vi "Begin.vi"() -> (0 "error out":errorcluster)   [LabVIEW 2013]
doc: "Called before other user functions, this VI is expected to open initial I/O refnums, load in file data, and do all program initialization. Notice that the <B>error out</B> terminal is simply used for data flow. Wiring it to other structures or subVIs ensures that this VI runs first."
uses:
  <vilib>/Rock Robotics/WPI/Camera/WPI_CameraImageSize.ctl
  <vilib>/Rock Robotics/SystemInterfaces/DIO/FPGA_DIOPWMChannel.ctl
  <vilib>/Rock Robotics/WPI/SafetyOutput/WPI_SafetyOutputConfigMenu.ctl
  <vilib>/Rock Robotics/WPI/Joystick/WPI_JoystickDeviceEnum.ctl
  <vilib>/Rock Robotics/SystemInterfaces/DIO/FPGA_DIOChannel.ctl
  <vilib>/Rock Robotics/SystemInterfaces/Typedef/FPGA_TypedefAnalogModule.ctl
  <vilib>/Rock Robotics/SystemInterfaces/AI/FPGA_AIChannel.ctl
  <vilib>/Rock Robotics/SystemInterfaces/Typedef/FPGA_TypedefSolenoidModule.ctl
  <vilib>/Rock Robotics/WPI/Solenoid/WPI_SolenoidChannel.ctl
  <vilib>/Rock Robotics/WPI/Solenoid/WPI_SolenoidValue.ctl
  <vilib>/Rock Robotics/SystemInterfaces/Typedef/FPGA_TypedefDigitalModule.ctl
  <vilib>/Rock Robotics/SystemInterfaces/DIO/FPGA_DIORelayChannel.ctl
  <vilib>/Rock Robotics/WPI/Relay/WPI_RelayValue.ctl
  <vilib>/Rock Robotics/WPI/Relay/WPI_RelayDirection.ctl
  <vilib>/Rock Robotics/SystemInterfaces/Typedef/FPGA_TypedefAnalogModuleForGyro.ctl
  <vilib>/Rock Robotics/SystemInterfaces/AI/FPGA_AIGyroChannel.ctl
  <vilib>/Rock Robotics/WPI/DriverStation/WPI_DriverStationRobotMode2.ctl
  <vilib>/Rock Robotics/WPI/RobotDrive/WPI_RobotDriveOpen2MotorWithTalon.vi
  <vilib>/Rock Robotics/WPI/Counter/WPI_CounterDigitalInputToDigitalSource.vi
  <vilib>/Rock Robotics/WPI/Solenoid/WPI_SolenoidOpenDouble.vi
  <vilib>/Rock Robotics/WPI/Solenoid/WPI_SolenoidSetEnum.vi
  <vilib>/Rock Robotics/WPI/MotorControl/WPI_MotorControlOpen Victor.vi
  <vilib>/Rock Robotics/WPI/MotorControl/WPI_MotorControlOpen Talon.vi
  <vilib>/Rock Robotics/WPI/Counter/WPI_CounterOpen Gear Tooth Sensor Mode.vi
  Robot Global Data.vi
  <vilib>/Rock Robotics/WPI/Camera/WPI_CameraWhite Balance Values.ctl
  <vilib>/Rock Robotics/WPI/Camera/WPI_CameraExposure Values.ctl
  <vilib>/Rock Robotics/WPI/Camera/WPI_CameraFrameRate.ctl
  <vilib>/Rock Robotics/WPI/Counter/WPI_CounterOpen UpDown Mode.vi
  <vilib>/Rock Robotics/WPI/Solenoid/WPI_SolenoidOpenSingle.vi
panel:
  out "created new? axes":bool
  out "created new?":bool
  in  "Image Size":T1=enum."160x120"
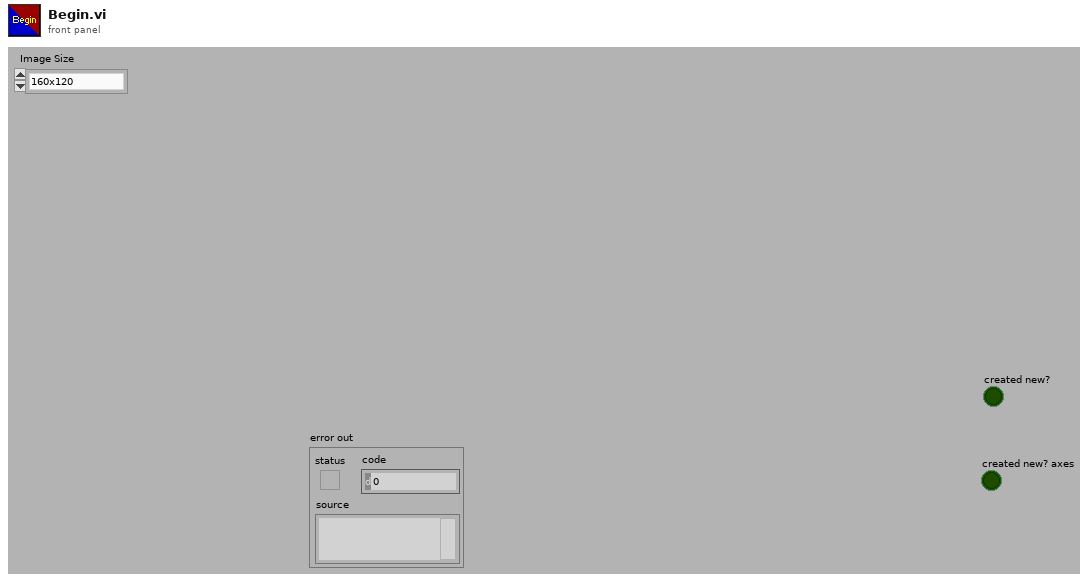
[diagram p1: front panel]
types:
  T1 = typedef "WPI_CameraImageSize.ctl" = enum16{"640x480", "320x240", "160x120"}
  T2 = typedef "WPI_DriverStationRobotMode2.ctl" = enum16{"Autonomous Disabled", "Autonomous Enabled", "Teleop Disabled", "Teleop Enabled", "Timeout", "Finish", "Test Disabled", "Test Enabled"}
  T3 = typedef "FPGA_AIChannel.ctl" = enum8{"AI 1", "AI 2", "AI 3", "AI 4", "AI 5", "AI 6", "AI 7", "AI 8", "Invalid"}
  T4 = typedef "FPGA_TypedefAnalogModule.ctl" = enum16{"Analog Module 1", "Analog Module 2"}
  T5 = typedef "FPGA_DIOPWMChannel.ctl" = enum8{"PWM 1", "PWM 2", "PWM 3", "PWM 4", "PWM 5", "PWM 6", "PWM 7", "PWM 8", "PWM 9", "PWM 10", "Invalid"}
  T6 = typedef "FPGA_TypedefDigitalModule.ctl" = enum16{"Digital Module 1", "Digital Module 2"}
  T7 = typedef "WPI_SolenoidValue.ctl" = enum16{"Off", "On", "Forward", "Reverse"}
  T8 = typedef "WPI_SolenoidChannel.ctl" = enum8{"Solenoid 1", "Solenoid 2", "Solenoid 3", "Solenoid 4", "Solenoid 5", "Solenoid 6", "Solenoid 7", "Solenoid 8", "Invalid"}
  T9 = typedef "FPGA_TypedefSolenoidModule.ctl" = enum16{"Solenoid Module 1", "Solenoid Module 2"}
  T10 = typedef "FPGA_DIOChannel.ctl" = enum8{"DIO 1", "DIO 2", "DIO 3", "DIO 4", "DIO 5", "DIO 6", "DIO 7", "DIO 8", "DIO 9", "DIO 10", "DIO 11", "DIO 12", "DIO 13", "DIO 14", "Invalid"}
  T11 = enum16{"open", "open or create", "create or replace", "create", "open (read-only)"}
  T12 = typedef "WPI_RelayDirection.ctl" = enum16{"Both directions", "Forward only", "Reverse only"}
  T13 = typedef "FPGA_DIORelayChannel.ctl" = enum8{"Relay 1", "Relay 2", "Relay 3", "Relay 4", "Relay 5", "Relay 6", "Relay 7", "Relay 8", "Invalid"}
  T14 = typedef "FPGA_AIGyroChannel.ctl" = enum8{"AI 1", "AI 2", "Invalid"}
  T15 = typedef "FPGA_TypedefAnalogModuleForGyro.ctl" = enum16{"Analog Module 1"}
  T16 = typedef "WPI_RelayValue.ctl" = enum16{"Off", "On", "Forward", "Reverse"}
  T17 = typedef "WPI_JoystickDeviceEnum.ctl" = enum16{"USB 1", "USB 2", "USB 3", "USB 4", "Kinect 1", "Kinect 2"}
  T18 = typedef "WPI_SafetyOutputConfigMenu.ctl" = enum16{"Enable", "Disable"}
  T19 = typedef "WPI_DigitalInputDevRef.ctl" = cluster{"DevStatus":errorcluster, "DIO Channel":T10, "Digital Module":T6}
  T20 = typedef "WPI_JoystickDevRef.ctl" = cluster{"Device":T17}
  T21 = typedef "WPI_RelayDevRef.ctl" = cluster{"DevStatus":errorcluster, "Relay Channel":T13, "Digital Module":T6, "Relay Direction":T12}
  T22 = enum16{"Rising Edge", "Falling Edge", "Raising & Falling Edge", "Disabled"}
  T23 = typedef "FPGA_CounterEncoderSourceConvertionLVSourceType.ctl" = cluster{"DevStatus":errorcluster, "AnalogTriggerMode?":bool, "DigitalMode":cluster{"Digital Module":T6, "DIO Channel":T24}, "AnalogTriggerMode":cluster{"AnalogTriggerIndex":T25, "OutputType":T26}}
  T24 = typedef "FPGA_DIODigitalSourceChannel.ctl" = enum8{"DIO 1", "DIO 2", "DIO 3", "DIO 4", "DIO 5", "DIO 6", "DIO 7", "DIO 8", "DIO 9", "DIO 10", "DIO 11", "DIO 12", "DIO 13", "DIO 14", "Disabled"}
  T25 = typedef "FPGA_AnalogTriggerIndex.ctl" = enum8{"Trig 0", "Trig 1", "Trig 2", "Trig 3", "Trig 4", "Trig 5", "Trig 6", "Trig 7", "Invalid"}
  T26 = typedef "FPGA_AnalogTriggerOutType.ctl" = enum16{"InWindow", "TriggerState", "Rising", "Falling"}
  T27 = typedef "WPI_CounterDevRef.ctl" = cluster{"DevStatus":errorcluster, "CntIndex":T28}
  T28 = typedef "FPGA_CounterCtrSystemIndex.ctl" = enum8{"Ctr 0", "Ctr 1", "Ctr 2", "Ctr 3", "Ctr 4", "Ctr 5", "Ctr 6", "Ctr 7", "Invalid"}
  T29 = typedef "WPI_ServoDeviceRef.ctl" = cluster{"DeviceStatus":errorcluster, "Digital Module":T6, "PWM Channel":T5, "DeadBand":T30}
  T30 = typedef "WPI_PWMDeadband.ctl" = cluster{"Name":string, "maxPositivePwm":i32, "minPositivePwm":i32, "centerPwm":i32, "maxNegativePwm":i32, "minNegativePwm":i32, "angularRange":u16}
  T31 = typedef "WPI_MotorControlDeviceRef.ctl" = cluster{"DeviceStatus":errorcluster, "Type":enum16{"PWM", "CAN"}, "PWM":cluster{"Digital Module":T6, "PWM Channel":T5, "DeadBand":T30}, "CAN":cluster{"Device Number":u8, "Control Mode":T32, "Semaphore":T33, "Max Vout":dbl}, "Invert":bool, "TransformRef":T34, "InvTransformRef":T34}
  T32 = typedef "WPI_CANJaguar_ControlMode.ctl" = enum8{"Percent VBus", "Current", "Speed", "Position", "Voltage"}
  T33 = typedef "Semaphore RefNum" = refnum<k1>
  T34 = typedef "WPI_PWMTransform_ConPane.ctl" = refnum<vi>
  T35 = typedef "WPI_SolenoidDevRef.ctl" = cluster{"DevStatus":errorcluster, "Solenoid Module":T9, "Forward Solenoid Channel":T8, "Reverse Solenoid Channel":T8}
  T36 = typedef "WPI_AnalogChannelDevRef.ctl" = cluster{"DevStatus":errorcluster, "Analog Module":T4, "Analog Channel":T3}
  T37 = typedef "WPI_RobotDriveDevRef.ctl" = cluster{"DevStatus":errorcluster, "Motors[]":T31[], "Square Inputs":bool, "Max Output":dbl, "Isochronous":bool}
  T38 = typedef "WPI_EncoderDevRef.ctl" = cluster{"DevStatus":errorcluster, "EncoderIndex":T39, "CounterIndex":T28, "DistancePerCount":dbl, "Decoding Type":T40}
  T39 = typedef "FPGA_EncoderIdx.ctl" = enum8{"Enc 0", "Enc 1", "Enc 2", "Enc 3", "Invalid"}
  T40 = typedef "WPI_EncoderType.ctl" = enum16{"1x", "2x", "4x"}
  T41 = typedef "WPI_GyroDevRef.ctl" = cluster{"DevStatus":errorcluster, "Analog Module":T4, "Analog Channel":T3, "Offset":dbl, "Gain (VoltsPerDegree/Second)":dbl}
  T42 = typedef "WPI_CameraFrameRate.ctl" = u32
  T43 = typedef "WPI_CameraExposure Values.ctl" = enum16{"Auto", "Flicker-free 50 Hz", "Flicker-free 60 Hz", "Hold current"}
  T44 = typedef "WPI_CameraWhite Balance Values.ctl" = enum16{"Auto", "Fixed indoor", "Fixed outdoor 1", "Fixed outdoor 2", "Fixed fluorescent 1", "Fixed fluorescent 2", "Hold current"}
  T45 = typedef "WPI_CameraDevRef.ctl" = cluster{"Camera Address":string, "CameraStatus":errorcluster, "Acquire Image Notifier":refnum<notifier>}
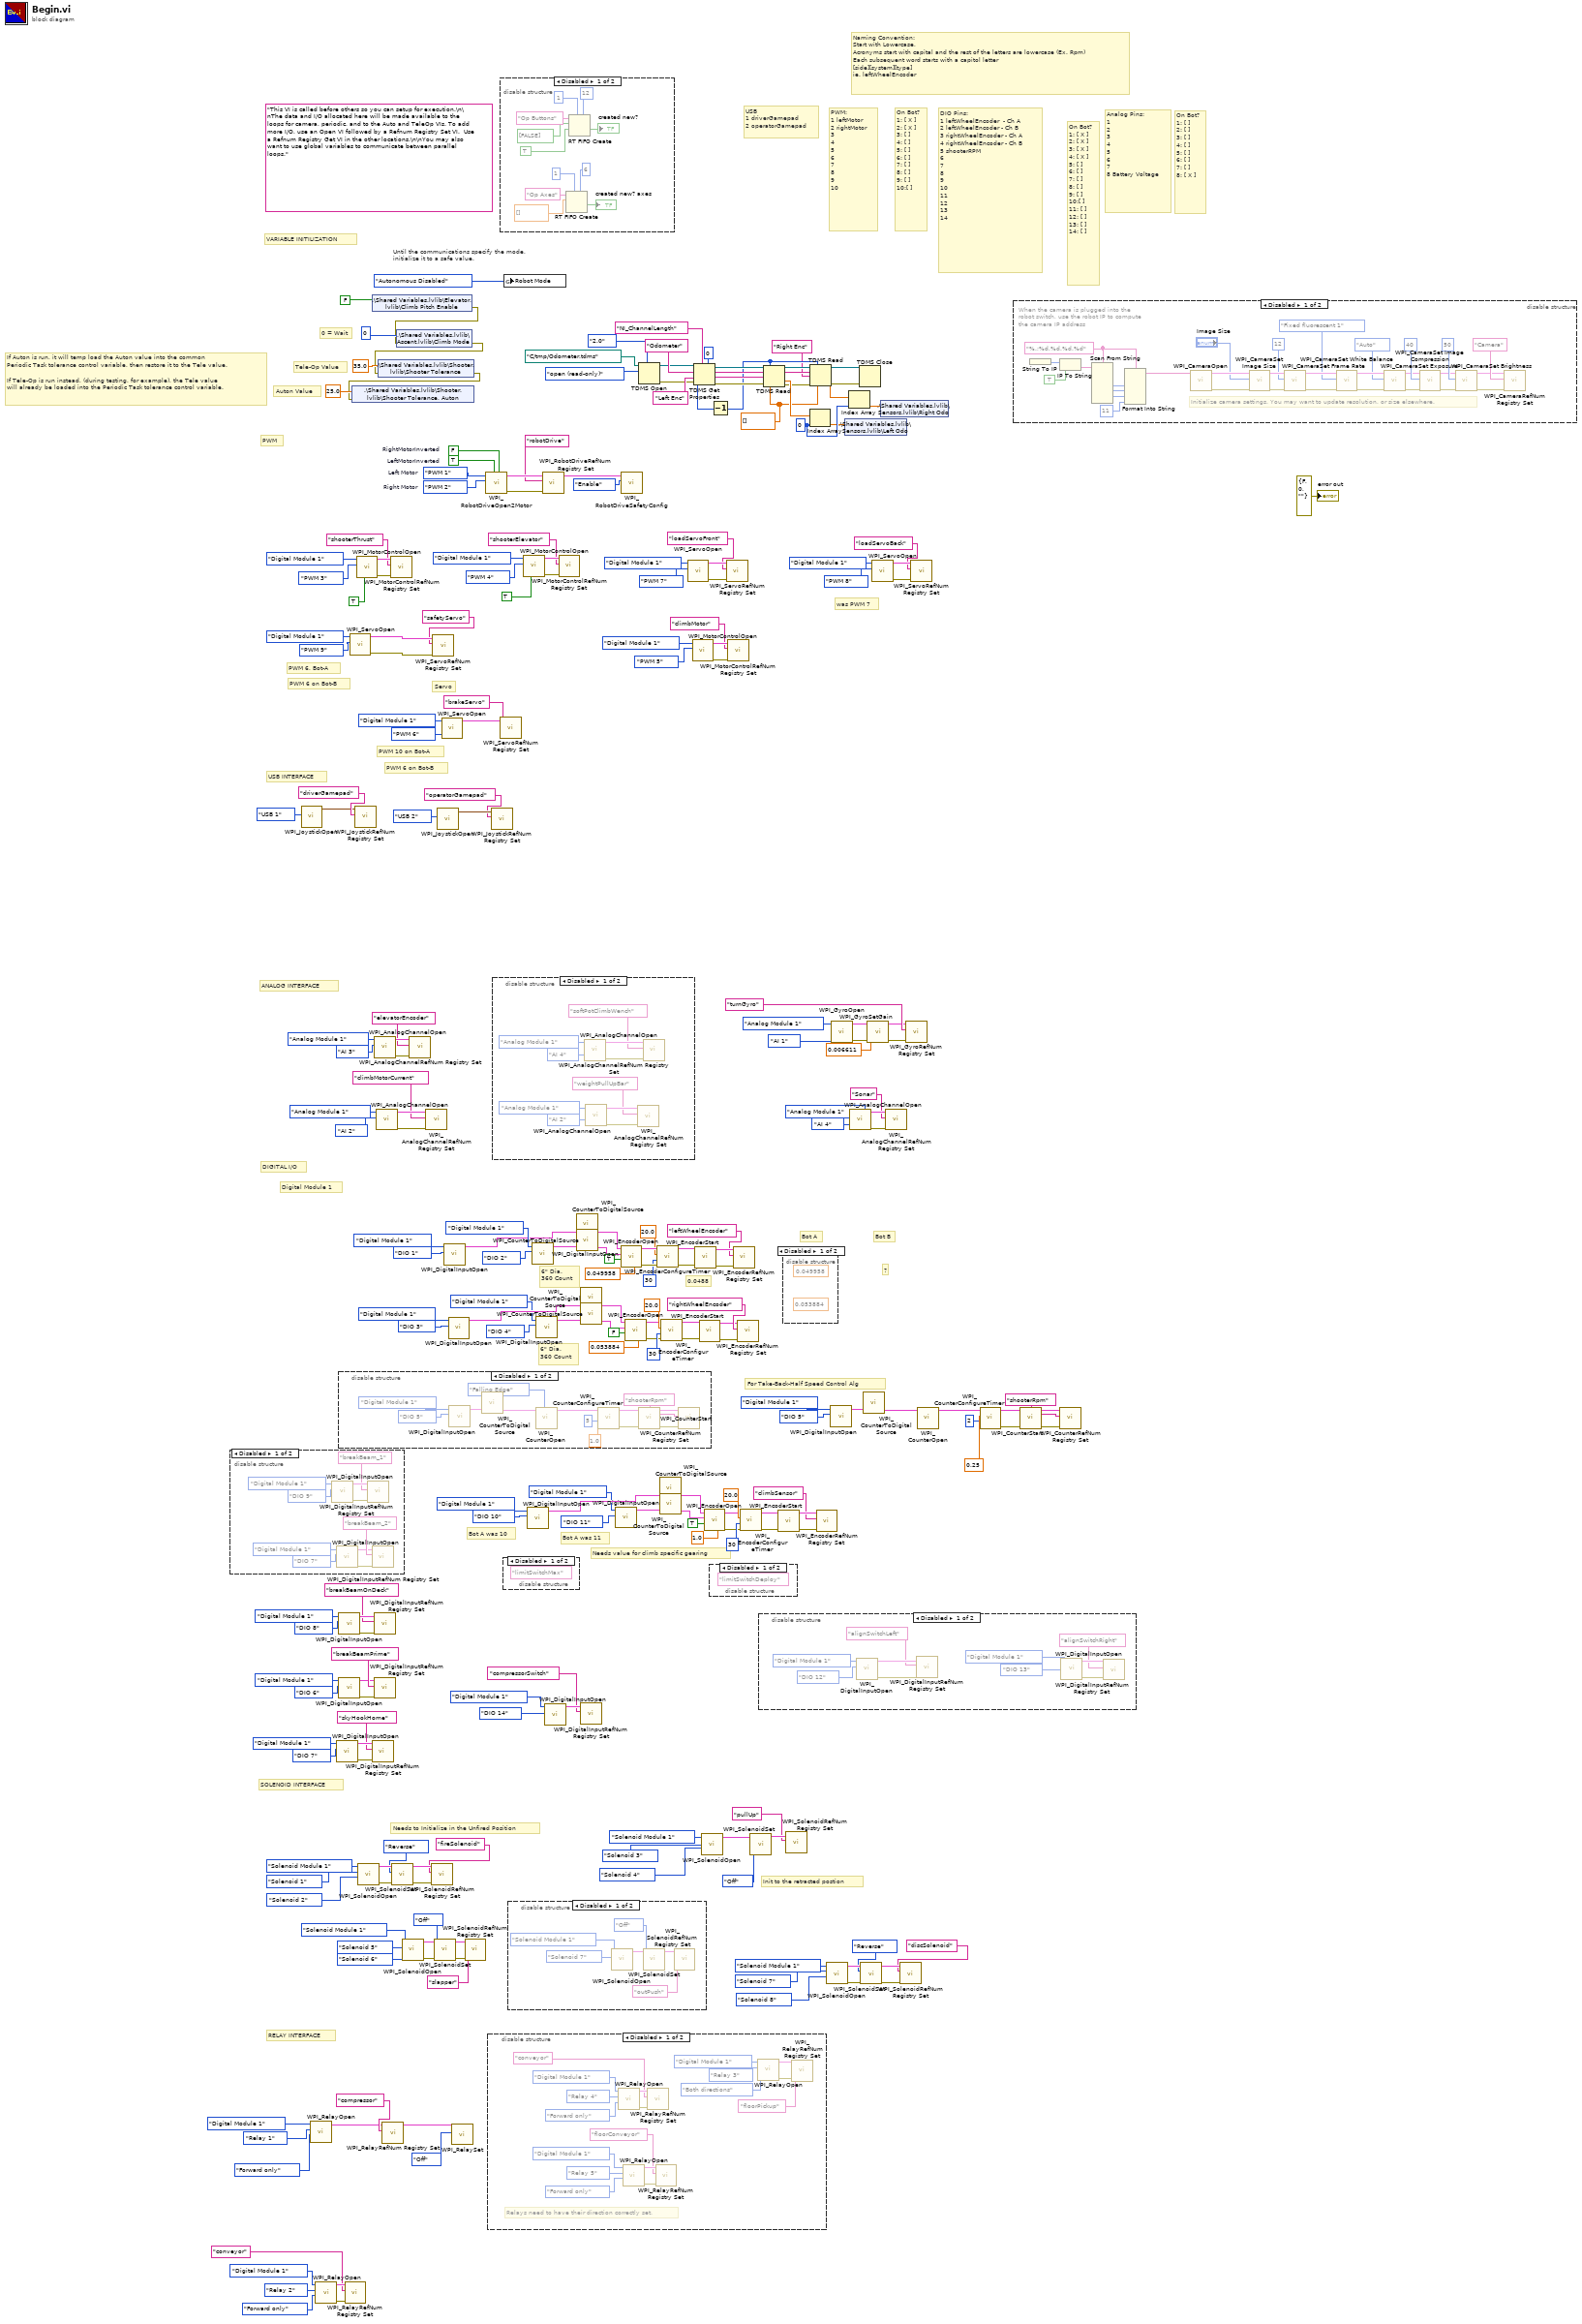
[diagram p0: block diagram]
diagram:
  w8 = 0 ("index")
  w12 = dbl[] []
  (unwired) "This VI is called before others so you can setup for execution.\n\nThe data and I/O allocated here will be made available to the loops for camera, periodic, and to the Auto and TeleOp VIs. To add more I/O, use an Open VI followed by a Refnum Registry Set VI.  Use a Refnum Registry Get VI in the other locations.\n\nYou may also want to use global variables to communicate between parallel loops."
  w239 = FPGA_DIOPWMChannel."PWM 2"  # Right Motor
  w240 = FPGA_DIOPWMChannel."PWM 1"  # Left Motor
  w244 = TRUE  # LeftMotorInverted
  w245 = FALSE  # RightMotorInverted
  # "If Auton is run, it will temp load the Auton value into the common\nPeriodic Task tolerance control variable, then restore it to the Tele value.\n\nIf Tele-Op is run instead, (during testing, for example), the Tele value\nwill already be loaded into the Periodic Task tolerance control variable."
  # "Auton Value"
  # "Tele-Op Value"
  # "Until the communications specify the mode,\ninitialize it to a safe value."
  # "0 = Wait"
  # "was PWM 7"
  # "PWM 10 on Bot-A"
  # "PWM 6 on Bot-B"
  # "PWM 6 on Bot-B"
  # "PWM 6, Bot-A"
  # "Servo"
  # "Bot A was 11"
  # "Bot A was 10"
  # "For Take-Back-Half Speed Control Alg"
  # "?"
  # "Bot B"
  # "Bot A"
  # "0.0488"
  # "Init to the retracted postion"
  # "Needs value for climb specific gearing"
  # "Needs to Initialize in the Unfired Position"
  # "Naming Convention:\nStart with Lowercase,\nAcronyms start with capital and the rest of the letters are lowercase (Ex. Rpm)\nEach subsequent word starts with a capitol letter\n[side][system][type]\nie. leftWheelEncoder"
  # "On Bot?\n1: [ ]\n2: [ ]\n3: [ ]\n4: [ ]\n5: [ ]\n6: [ ]\n7: [ ]\n8: [ X ]"
  # "On Bot?\n1: [ X ]\n2: [ X ]\n3: [ X ]\n4: [ X ]\n5: [ ]\n6: [ ]\n7: [ ]\n8: [ ]\n9: [ ]\n10:[ ]\n11: [ ]\n12: [ ]\n13: [ ]\n14: [ ]"
  # "On Bot?\n1: [ X ]\n2: [ X ]\n3: [ ]\n4: [ ]\n5: [ ]\n6: [ ]\n7: [ ]\n8: [ ]\n9: [ ]\n10:[ ]"
  # "6\" Dia. \n360 Count"
  # "6\" Dia. \n360 Count"
  # "PWM:\n1 leftMotor \n2 rightMotor\n3 \n4 \n5 \n6 \n7 \n8 \n9 \n10"
  # "USB\n1 driverGamepad\n2 operatorGamepad"
  # "Analog Pins:\n1 \n2 \n3 \n4 \n5 \n6 \n7 \n8 Battery Voltage"
  # "DIO Pins:\n1 leftWheelEncoder  - Ch A \n2 leftWheelEncoder - Ch B\n3 rightWheelEncoder - Ch A\n4 rightWheelEncoder - Ch B\n5 shooterRPM\n6  \n7 \n8 \n9 \n10 \n11 \n12 \n13 \n14"
  # "SOLENOID INTERFACE"
  # "Digital Module 1"
  # "DIGITAL I/O"
  # "ANALOG INTERFACE"
  # "RELAY INTERFACE"
  # "USB INTERFACE"
  # "VARIABLE INITILIZATION"
  # "PWM"
  n1 = disable-structure shown="Disabled" {
    frame Disabled {
      n2 = call <vilib>:"WPI_DigitalInputOpen.vi"("DIO Channel"=FPGA_DIOChannel."DIO 9", "Digital Module (Module 1)"=FPGA_TypedefDigitalModule."Digital Module 1") -> ("error out"=w255:errorcluster, "DigitalInputDevRef"=w254:T19)  [unwired: 8 in]
      n3 = call <vilib>:"WPI_DigitalInputOpen.vi"("DIO Channel"=FPGA_DIOChannel."DIO 7", "Digital Module (Module 1)"=FPGA_TypedefDigitalModule."Digital Module 1") -> ("error out"=w246:errorcluster, "DigitalInputDevRef"=w247:T19)  [unwired: 8 in]
      n4 = call <vilib>:"WPI_DigitalInputRefNum Registry Set.vi"("error in (no error)"=w255, "refnum name"="breakBeam_1", "DigitalInputDevRef"=w254) -> ()  [unwired: 7 in, 2 out]
      n5 = call <vilib>:"WPI_DigitalInputRefNum Registry Set.vi"("error in (no error)"=w246, "refnum name"="breakBeam_2", "DigitalInputDevRef"=w247) -> ()  [unwired: 7 in, 2 out]
    }
    frame Enabled {
    }
  }
  n6 = call <vilib>:"WPI_JoystickOpen.vi"("JoystickDevice"=WPI_JoystickDeviceEnum."USB 1") -> ("JoystickDevRef"=w235:T20)  [unwired: 10 in]
  n7 = call <vilib>:"WPI_RelayOpen.vi"("Relay Direction"=WPI_RelayDirection."Forward only", "Relay Channel"=FPGA_DIORelayChannel."Relay 1", "Digital Module (Module 1)"=FPGA_TypedefDigitalModule."Digital Module 1" ("Relay Digital Module (Module 1)")) -> ("RelayDevRef"=w100:T21)  [unwired: 7 in, 1 out]
  n8 = call <vilib>:"WPI_RelayOpen.vi"("Relay Direction"=WPI_RelayDirection."Forward only", "Relay Channel"=FPGA_DIORelayChannel."Relay 2", "Digital Module (Module 1)"=FPGA_TypedefDigitalModule."Digital Module 1") -> ("error out"=w86:errorcluster, "RelayDevRef"=w85:T21)  [unwired: 7 in]
  n9 = call <vilib>:"WPI_DigitalInputOpen.vi"("DIO Channel"=FPGA_DIOChannel."DIO 7", "Digital Module (Module 1)"=FPGA_TypedefDigitalModule."Digital Module 1") -> ("error out"=w55:errorcluster, "DigitalInputDevRef"=w54:T19)  [unwired: 8 in]
  n10 = disable-structure shown="Disabled" {
    frame Disabled {
      n11 = call <vilib>:"WPI_DigitalInputOpen.vi"("DIO Channel"=FPGA_DIOChannel."DIO 5", "Digital Module (Module 1)"=FPGA_TypedefDigitalModule."Digital Module 1") -> ("DigitalInputDevRef"=w268:T19)  [unwired: 8 in, 1 out]
      n12 = call-poly <vilib>:"WPI_CounterToDigitalSource.vi"("DigitalInputDevRef"=w268) -> ("Digital Source"=w267:T23)  [unwired: 6 in]
      n13 = call-poly <vilib>:"WPI_CounterOpen.vi"("UpEdge"=T22."Falling Edge", "Up Source"=w267) -> ("CounterDevRef"=w263:T27)  [unwired: 8 in, 1 out]
      n14 = call <vilib>:"WPI_CounterConfigureTimer.vi"("Number Samples to Average"=u8 5, "MaxPeriod (sec)"=1.0, "CounterDevRef in"=w263) -> ("error out"=w260:errorcluster, "CounterDevRef out"=w259:T27)  [unwired: 7 in]
      n15 = call <vilib>:"WPI_CounterStart.vi"("error in (no error)"=w260, "CounterDevRef in"=w259) -> ("error out"=w258:errorcluster, "CounterDevRef out"=w257:T27)  [unwired: 8 in]
      n16 = call <vilib>:"WPI_CounterRefNum Registry Set.vi"("error in (no error)"=w258, "refnum name"="shooterRpm", "CounterDevRef"=w257) -> ()  [unwired: 7 in, 2 out]
    }
    frame Enabled {
    }
  }
  n17 = call <vilib>:"WPI_DigitalInputOpen.vi"("DIO Channel"=FPGA_DIOChannel."DIO 8", "Digital Module (Module 1)"=FPGA_TypedefDigitalModule."Digital Module 1") -> ("error out"=w186:errorcluster, "DigitalInputDevRef"=w185:T19)  [unwired: 8 in]
  n18 = call <vilib>:"WPI_DigitalInputOpen.vi"("DIO Channel"=FPGA_DIOChannel."DIO 6", "Digital Module (Module 1)"=FPGA_TypedefDigitalModule."Digital Module 1") -> ("error out"=w177:errorcluster, "DigitalInputDevRef"=w178:T19)  [unwired: 8 in]
  n19 = call <vilib>:"WPI_RelayRefNum Registry Set.vi"("error in (no error)"=w86, "refnum name"="conveyor", "RelayDevRef"=w85) -> ()  [unwired: 7 in, 2 out]
  n20 = call <vilib>:"WPI_ServoOpen.vi"("PWM Channel"=FPGA_DIOPWMChannel."PWM 9", "Digital Module (Module 1)"=FPGA_TypedefDigitalModule."Digital Module 1") -> ("error out"=w161:errorcluster, "ServoDeviceRef"=w162:T29)  [unwired: 8 in]
  n21 = call <vilib>:"WPI_JoystickRefNum Registry Set.vi"("refnum name"="driverGamepad", "JoystickDevRef"=w235) -> ()  [unwired: 8 in, 2 out]
  n22 = call-poly <vilib>:"WPI_MotorControlOpen.vi"("Invert"=TRUE, "PWM Channel"=FPGA_DIOPWMChannel."PWM 3", "Digital Module (Module 1)"=FPGA_TypedefDigitalModule."Digital Module 1") -> ("error out"=w156:errorcluster, "MotorControlDeviceRef"=w157:T31)  [unwired: 7 in]
  n23 = call-poly <vilib>:"WPI_SolenoidOpen.vi"("Reverse Solenoid Channel"=WPI_SolenoidChannel."Solenoid 2", "Forward Solenoid Channel"=WPI_SolenoidChannel."Solenoid 1", "Solenoid Module (Module 1)"=FPGA_TypedefSolenoidModule."Solenoid Module 1") -> ("error out"=w173:errorcluster, "SolenoidDevRef"=w172:T35)  [unwired: 7 in]
  n24 = call <vilib>:"WPI_DigitalInputRefNum Registry Set.vi"("error in (no error)"=w55, "refnum name"="skyHookHome", "DigitalInputDevRef"=w54) -> ()  [unwired: 7 in, 2 out]
  n25 = shared-variable ".\\Shared Variables.lvlib\\Elevator.lvlib\\Climb Pitch Enable"(FALSE ("Climb Pitch Enable")) -> (error out=w5:errorcluster)  [unwired: 1 in]
  n26 = call <vilib>:"WPI_AnalogChannelOpen.vi"("Analog Channel"=FPGA_AIChannel."AI 3", "Analog Module (Module 1)"=FPGA_TypedefAnalogModule."Analog Module 1") -> ("error out"=w189:errorcluster, "AIDeviceRef"=w188:T36)  [unwired: 8 in]
  n27 = call <vilib>:"WPI_DigitalInputRefNum Registry Set.vi"("error in (no error)"=w186, "refnum name"="breakBeamOnDeck", "DigitalInputDevRef"=w185) -> ()  [unwired: 7 in, 2 out]
  n28 = call <vilib>:"WPI_DigitalInputRefNum Registry Set.vi"("error in (no error)"=w177, "refnum name"="breakBeamPrime", "DigitalInputDevRef"=w178) -> ()  [unwired: 7 in, 2 out]
  n29 = call <vilib>:"WPI_AnalogChannelOpen.vi"("Analog Channel"=FPGA_AIChannel."AI 2", "Analog Module (Module 1)"=FPGA_TypedefAnalogModule."Analog Module 1") -> ("error out"=w146:errorcluster, "AIDeviceRef"=w147:T36)  [unwired: 8 in]
  n30 = call <vilib>:"WPI_RelayRefNum Registry Set.vi"("refnum name"="compressor", "RelayDevRef"=w100) -> ("RelayDevRef"=w99:T21)  [unwired: 8 in, 1 out]
  n31 = call <vilib>:"WPI_MotorControlRefNum Registry Set.vi"("error in (no error)"=w156, "refnum name"="shooterThrust", "MotorControlDevRef"=w157) -> ()  [unwired: 7 in, 2 out]
  n32 = call-poly <vilib>:"WPI_SolenoidSet.vi"("error in (no error)"=w173, "Value"=WPI_SolenoidValue."Reverse", "SolenoidDevRef"=w172) -> ("error out"=w170:errorcluster, "SolenoidDevRef"=w169:T35)  [unwired: 7 in]
  n33 = shared-variable ".\\Shared Variables.lvlib\\Ascent.lvlib\\Climb Mode"(u16 0 ("Climb Mode"), error in=w5) -> (error out=w2:errorcluster)
  n34 = shared-variable ".\\Shared Variables.lvlib\\Shooter.lvlib\\Shooter Tolerance"(35.0 ("Shooter Tolerance"), error in=w2) -> (error out=w1:errorcluster)
  n35 = shared-variable ".\\Shared Variables.lvlib\\Shooter.lvlib\\Shooter Tolerance, Auton"(25.0 ("Shooter Tolerance, Auton"), error in=w1) -> ()  [unwired: 1 out]
  n36 = call-poly <vilib>:"WPI_SolenoidOpen.vi"("Reverse Solenoid Channel"=WPI_SolenoidChannel."Solenoid 6", "Forward Solenoid Channel"=WPI_SolenoidChannel."Solenoid 5", "Solenoid Module (Module 1)"=FPGA_TypedefSolenoidModule."Solenoid Module 1") -> ("error out"=w142:errorcluster, "SolenoidDevRef"=w141:T35)  [unwired: 7 in]
  n37 = call <vilib>:"WPI_AnalogChannelRefNum Registry Set.vi"("error in (no error)"=w189, "refnum name"="elevatorEncoder", "AIDeviceRef"=w188) -> ()  [unwired: 7 in, 2 out]
  n38 = call <vilib>:"WPI_AnalogChannelRefNum Registry Set.vi"("error in (no error)"=w146, "refnum name"="climbMotorCurrent", "AIDeviceRef"=w147) -> ()  [unwired: 7 in, 2 out]
  n39 = call <vilib>:"WPI_SolenoidRefNum Registry Set.vi"("error in (no error)"=w170, "refnum name"="fireSolenoid", "SolenoidDevRef"=w169) -> ()  [unwired: 7 in, 2 out]
  n40 = call <vilib>:"WPI_ServoRefNum Registry Set.vi"("error in (no error)"=w161, "refnum name"="safetyServo", "ServoDeviceRef"=w162) -> ()  [unwired: 7 in, 2 out]
  n41 = call-poly <vilib>:"WPI_SolenoidSet.vi"("error in (no error)"=w142, "Value"=WPI_SolenoidValue."Off", "SolenoidDevRef"=w141) -> ("error out"=w140:errorcluster, "SolenoidDevRef"=w139:T35)  [unwired: 7 in]
  n42 = call <vilib>:"WPI_JoystickOpen.vi"("JoystickDevice"=WPI_JoystickDeviceEnum."USB 2") -> ("JoystickDevRef"=w194:T20)  [unwired: 10 in]
  n43 = call <vilib>:"WPI_ServoOpen.vi"("PWM Channel"=FPGA_DIOPWMChannel."PWM 6", "Digital Module (Module 1)"=FPGA_TypedefDigitalModule."Digital Module 1") -> ("ServoDeviceRef"=w27:T29)  [unwired: 8 in, 1 out]
  n44 = call <vilib>:"WPI_DigitalInputOpen.vi"("DIO Channel"=FPGA_DIOChannel."DIO 1", "Digital Module (Module 1)"=FPGA_TypedefDigitalModule."Digital Module 1") -> ("DigitalInputDevRef"=w228:T19)  [unwired: 8 in, 1 out]
  n45 = call <vilib>:"WPI_DigitalInputOpen.vi"("DIO Channel"=FPGA_DIOChannel."DIO 3", "Digital Module (Module 1)"=FPGA_TypedefDigitalModule."Digital Module 1") -> ("DigitalInputDevRef"=w201:T19)  [unwired: 8 in, 1 out]
  n46 = call <vilib>:"WPI_RelaySet.vi"("RelayValue"=WPI_RelayValue."Off", "RelayDevRef"=w99) -> ()  [unwired: 8 in, 2 out]
  n47 = call <vilib>:"WPI_SolenoidRefNum Registry Set.vi"("error in (no error)"=w140, "refnum name"="slapper", "SolenoidDevRef"=w139) -> ()  [unwired: 7 in, 2 out]
  n48 = call-poly <vilib>:"WPI_RobotDriveOpen2Motor.vi"("Right Motor Inverted"=w245, "Left Motor Inverted"=w244, "Right Motor"=w239, "Left Motor"=w240) -> ("error out"=w241:errorcluster, "RobotDriveDevRef"=w243:T37)  [unwired: 6 in]
  n49 = disable-structure shown="Disabled" {
    frame Disabled {
      # "Relays need to have their direction correctly set."
      n50 = call <vilib>:"WPI_RelayOpen.vi"("Relay Direction"=WPI_RelayDirection."Forward only", "Relay Channel"=FPGA_DIORelayChannel."Relay 4", "Digital Module (Module 1)"=FPGA_TypedefDigitalModule."Digital Module 1") -> ("error out"=w286:errorcluster, "RelayDevRef"=w285:T21)  [unwired: 7 in]
      n51 = call <vilib>:"WPI_RelayOpen.vi"("Relay Direction"=WPI_RelayDirection."Forward only", "Relay Channel"=FPGA_DIORelayChannel."Relay 5", "Digital Module (Module 1)"=FPGA_TypedefDigitalModule."Digital Module 1") -> ("error out"=w280:errorcluster, "RelayDevRef"=w279:T21)  [unwired: 7 in]
      n52 = call <vilib>:"WPI_RelayRefNum Registry Set.vi"("error in (no error)"=w286, "refnum name"="conveyor", "RelayDevRef"=w285) -> ()  [unwired: 7 in, 2 out]
      n53 = call <vilib>:"WPI_RelayRefNum Registry Set.vi"("error in (no error)"=w280, "refnum name"="floorConveyor", "RelayDevRef"=w279) -> ()  [unwired: 7 in, 2 out]
      n54 = call <vilib>:"WPI_RelayOpen.vi"("Relay Direction"=WPI_RelayDirection."Both directions", "Relay Channel"=FPGA_DIORelayChannel."Relay 3", "Digital Module (Module 1)"=FPGA_TypedefDigitalModule."Digital Module 1") -> ("error out"=w273:errorcluster, "RelayDevRef"=w274:T21)  [unwired: 7 in]
      n55 = call <vilib>:"WPI_RelayRefNum Registry Set.vi"("error in (no error)"=w273, "refnum name"="floorPickup", "RelayDevRef"=w274) -> ()  [unwired: 7 in, 2 out]
    }
    frame Enabled {
    }
  }
  n56 = call <vilib>:"WPI_JoystickRefNum Registry Set.vi"("refnum name"="operatorGamepad", "JoystickDevRef"=w194) -> ()  [unwired: 8 in, 2 out]
  n57 = disable-structure shown="Disabled" {
    frame Disabled {
      n58 = call <vilib>:"WPI_AnalogChannelOpen.vi"("Analog Channel"=FPGA_AIChannel."AI 4", "Analog Module (Module 1)"=FPGA_TypedefAnalogModule."Analog Module 1") -> ("error out"=w295:errorcluster, "AIDeviceRef"=w296:T36)  [unwired: 8 in]
      n59 = call <vilib>:"WPI_AnalogChannelOpen.vi"("Analog Channel"=FPGA_AIChannel."AI 2", "Analog Module (Module 1)"=FPGA_TypedefAnalogModule."Analog Module 1") -> ("error out"=w293:errorcluster, "AIDeviceRef"=w294:T36)  [unwired: 8 in]
      n60 = call <vilib>:"WPI_AnalogChannelRefNum Registry Set.vi"("error in (no error)"=w293, "refnum name"="weightPullUpBar", "AIDeviceRef"=w294) -> ()  [unwired: 7 in, 2 out]
      n61 = call <vilib>:"WPI_AnalogChannelRefNum Registry Set.vi"("error in (no error)"=w295, "refnum name"="softPotClimbWench", "AIDeviceRef"=w296) -> ()  [unwired: 7 in, 2 out]
    }
    frame Enabled {
    }
  }
  n62 = disable-structure shown="Disabled" {
    frame Disabled {
      n63 = RT FIFO Create(0:"Op Axes" ("name (unnamed)"), 1:dbl[] [], 4:u32 1 ("size (10)"), 6:u32 6 ("elements in array (1)")) -> (10:→"created new? axes":bool)  [unwired: 4 in, 2 out]
      n64 = RT FIFO Create(0:"Op Buttons" ("name (unnamed)"), 1:bool[] [FALSE], 2:TRUE ("create if not found? (T)"), 4:u32 1 ("size (10)"), 6:u32 12 ("elements in array (1)")) -> (10:→"created new?":bool)  [unwired: 3 in, 2 out]
    }
    frame Enabled {
    }
  }
  n65 = call <vilib>:"WPI_ServoRefNum Registry Set.vi"("refnum name"="brakeServo", "ServoDeviceRef"=w27) -> ()  [unwired: 8 in, 2 out]
  n66 = disable-structure shown="Disabled" {
    frame Disabled {
      (unwired) "limitSwitchMax" ("refnum name")
    }
    frame Enabled {
    }
  }
  n67 = global write "Robot Global Data.vi" "Robot Mode"(WPI_DriverStationRobotMode2."Autonomous Disabled" ("Robot Mode")) -> ()
  n68 = disable-structure shown="Disabled" {
    frame Disabled {
      n69 = call-poly <vilib>:"WPI_SolenoidOpen.vi"("Solenoid Channel"=WPI_SolenoidChannel."Solenoid 7" ("Forward Solenoid Channel"), "Solenoid Module (Module 1)"=FPGA_TypedefSolenoidModule."Solenoid Module 1") -> ("SolenoidDevRef"=w313:T35)  [unwired: 8 in, 1 out]
      n70 = call-poly <vilib>:"WPI_SolenoidSet.vi"("Value"=WPI_SolenoidValue."Off", "SolenoidDevRef"=w313) -> ("SolenoidDevRef"=w312:T35)  [unwired: 8 in, 1 out]
      n71 = call <vilib>:"WPI_SolenoidRefNum Registry Set.vi"("refnum name"="outPush", "SolenoidDevRef"=w312) -> ()  [unwired: 8 in, 2 out]
    }
    frame Enabled {
    }
  }
  n72 = call-poly <vilib>:"WPI_MotorControlOpen.vi"("Invert"=TRUE, "PWM Channel"=FPGA_DIOPWMChannel."PWM 4", "Digital Module (Module 1)"=FPGA_TypedefDigitalModule."Digital Module 1") -> ("error out"=w154:errorcluster, "MotorControlDeviceRef"=w155:T31)  [unwired: 7 in]
  n73 = call <vilib>:"WPI_DigitalInputOpen.vi"("DIO Channel"=FPGA_DIOChannel."DIO 10", "Digital Module (Module 1)"=FPGA_TypedefDigitalModule."Digital Module 1") -> ("DigitalInputDevRef"=w122:T19)  [unwired: 8 in, 1 out]
  n74 = call <vilib>:"WPI_DigitalInputOpen.vi"("DIO Channel"=FPGA_DIOChannel."DIO 2", "Digital Module (Module 1)"=FPGA_TypedefDigitalModule."Digital Module 1") -> ("DigitalInputDevRef"=w229:T19)  [unwired: 8 in, 1 out]
  n75 = call <vilib>:"WPI_DigitalInputOpen.vi"("DIO Channel"=FPGA_DIOChannel."DIO 4", "Digital Module (Module 1)"=FPGA_TypedefDigitalModule."Digital Module 1") -> ("DigitalInputDevRef"=w200:T19)  [unwired: 8 in, 1 out]
  n76 = call <vilib>:"WPI_RobotDriveRefNum Registry Set.vi"("error in (no error)"=w241, "refnum name"="robotDrive", "RobotDriveDevRef"=w243) -> ("RobotDriveDevRef"=w238:T37)  [unwired: 8 out]
  n77 = call <vilib>:"WPI_DigitalInputOpen.vi"("DIO Channel"=FPGA_DIOChannel."DIO 14" ("Pressure Switch DIO Channel"), "Digital Module (Module 1)"=FPGA_TypedefDigitalModule."Digital Module 1" ("Pressure Switch Digital Module (Module 1)")) -> ("DigitalInputDevRef"=w92:T19)  [unwired: 8 in, 1 out]
  n78 = call <vilib>:"WPI_MotorControlRefNum Registry Set.vi"("error in (no error)"=w154, "refnum name"="shooterElevator", "MotorControlDevRef"=w155) -> ()  [unwired: 7 in, 2 out]
  n79 = call-poly <vilib>:"WPI_CounterToDigitalSource.vi"("DigitalInputDevRef"=w228) -> ("Digital Source"=w227:T23)  [unwired: 6 in]
  n80 = call-poly <vilib>:"WPI_CounterToDigitalSource.vi"("DigitalInputDevRef"=w229) -> ("Digital Source"=w226:T23)  [unwired: 6 in]
  n81 = call-poly <vilib>:"WPI_CounterToDigitalSource.vi"("DigitalInputDevRef"=w201) -> ("Digital Source"=w202:T23)  [unwired: 6 in]
  n82 = call-poly <vilib>:"WPI_CounterToDigitalSource.vi"("DigitalInputDevRef"=w200) -> ("Digital Source"=w203:T23)  [unwired: 6 in]
  n83 = call <vilib>:"WPI_DigitalInputRefNum Registry Set.vi"("refnum name"="compressorSwitch", "DigitalInputDevRef"=w92) -> ()  [unwired: 8 in, 2 out]
  n84 = call <vilib>:"WPI_DigitalInputOpen.vi"("DIO Channel"=FPGA_DIOChannel."DIO 11", "Digital Module (Module 1)"=FPGA_TypedefDigitalModule."Digital Module 1") -> ("DigitalInputDevRef"=w121:T19)  [unwired: 8 in, 1 out]
  n85 = call <vilib>:"WPI_EncoderOpen.vi"("DistancePerCount"=0.049958, "Invert Direction (False)"=TRUE, "BSource"=w226, "ASource"=w227) -> ("error out"=w223:errorcluster, "EncoderDevRef"=w222:T38)  [unwired: 6 in]
  n86 = call <vilib>:"WPI_RobotDriveSafetyConfig.vi"("mode"=WPI_SafetyOutputConfigMenu."Enable", "RobotDriveDevRef"=w238) -> ()  [unwired: 8 in, 2 out]
  n87 = call <vilib>:"WPI_EncoderOpen.vi"("DistancePerCount"=0.053884, "Invert Direction (False)"=FALSE, "BSource"=w203, "ASource"=w202) -> ("error out"=w206:errorcluster, "EncoderDevRef"=w207:T38)  [unwired: 6 in]
  n88 = TDMS Open(7:enum16{"1.0", "2.0"}."2.0" ("file format version (2.0)"), 10:T11."open (read-only)" ("operation (0:open)"), 11:path "C:/tmp/Odometer.tdms" ("file path")) -> (0:w67:errorcluster, 3:w65:refnum<k34>)  [unwired: 4 in]
  n89 = call <vilib>:"WPI_EncoderConfigureTimer.vi"("error in (no error)"=w223, "Number Samples to Average"=u8 30, "Minimum Rate"=20.0, "EncoderDevRef"=w222) -> ("error out"=w219:errorcluster, "EncoderDevRef"=w218:T38)  [unwired: 6 in]
  n90 = call-poly <vilib>:"WPI_CounterToDigitalSource.vi"("DigitalInputDevRef"=w122) -> ("Digital Source"=w123:T23)  [unwired: 6 in]
  n91 = call-poly <vilib>:"WPI_CounterToDigitalSource.vi"("DigitalInputDevRef"=w121) -> ("Digital Source"=w124:T23)  [unwired: 6 in]
  n92 = call <vilib>:"WPI_EncoderConfigureTimer.vi"("error in (no error)"=w206, "Number Samples to Average"=u8 30, "Minimum Rate"=20.0, "EncoderDevRef"=w207) -> ("error out"=w210:errorcluster, "EncoderDevRef"=w211:T38)  [unwired: 6 in]
  n93 = call <vilib>:"WPI_ServoOpen.vi"("PWM Channel"=FPGA_DIOPWMChannel."PWM 7", "Digital Module (Module 1)"=FPGA_TypedefDigitalModule."Digital Module 1") -> ("error out"=w167:errorcluster, "ServoDeviceRef"=w166:T29)  [unwired: 8 in]
  n94 = call-poly <vilib>:"WPI_MotorControlOpen.vi"("PWM Channel"=FPGA_DIOPWMChannel."PWM 5", "Digital Module (Module 1)"=FPGA_TypedefDigitalModule."Digital Module 1") -> ("error out"=w114:errorcluster, "MotorControlDeviceRef"=w115:T31)  [unwired: 8 in]
  n95 = TDMS Get Properties(5:0, 7:"NI_ChannelLength" ("property name"), 8:w67, 9:"Left Enc" ("channel name"), 10:"Odometer" ("group name"), 11:w65) -> (0:w66:errorcluster, 1:w70:string, 2:w71:string, 3:w69:refnum<k34>, 4:w64:i32)  [unwired: 1 out]
  n96 = call <vilib>:"WPI_EncoderStart.vi"("error in (no error)"=w219, "EncoderDevRef"=w218) -> ("error out"=w217:errorcluster, "EncoderDevRef"=w216:T38)  [unwired: 8 in]
  n97 = call <vilib>:"WPI_EncoderStart.vi"("error in (no error)"=w210, "EncoderDevRef"=w211) -> ("error out"=w212:errorcluster, "EncoderDevRef"=w213:T38)  [unwired: 8 in]
  n98 = call-poly <vilib>:"WPI_SolenoidOpen.vi"("Reverse Solenoid Channel"=WPI_SolenoidChannel."Solenoid 4", "Forward Solenoid Channel"=WPI_SolenoidChannel."Solenoid 3", "Solenoid Module (Module 1)"=FPGA_TypedefSolenoidModule."Solenoid Module 1") -> ("SolenoidDevRef"=w108:T35)  [unwired: 7 in, 1 out]
  n99 = call <vilib>:"WPI_EncoderOpen.vi"("DistancePerCount"=1.0, "Invert Direction (False)"=TRUE, "BSource"=w124, "ASource"=w123) -> ("error out"=w127:errorcluster, "EncoderDevRef"=w128:T38)  [unwired: 6 in]
  n100 = disable-structure shown="Disabled" {
    frame Disabled {
      (unwired) "limitSwitchDeploy" ("refnum name")
    }
    frame Enabled {
    }
  }
  n101 = Decrement(x=w64) -> (x-1=w63:i32)
  n102 = call <vilib>:"WPI_ServoRefNum Registry Set.vi"("error in (no error)"=w167, "refnum name"="loadServoFront", "ServoDeviceRef"=w166) -> ()  [unwired: 7 in, 2 out]
  n103 = call <vilib>:"WPI_MotorControlRefNum Registry Set.vi"("error in (no error)"=w114, "refnum name"="climbMotor", "MotorControlDevRef"=w115) -> ()  [unwired: 7 in, 2 out]
  n104 = call <vilib>:"WPI_EncoderRefNum Registry Set.vi"("error in (no error)"=w217, "refnum name"="leftWheelEncoder", "EncoderDevRef"=w216) -> ()  [unwired: 7 in, 2 out]
  n105 = call <vilib>:"WPI_EncoderRefNum Registry Set.vi"("error in (no error)"=w212, "refnum name"="rightWheelEncoder", "EncoderDevRef"=w213) -> ()  [unwired: 7 in, 2 out]
  n106 = call <vilib>:"WPI_EncoderConfigureTimer.vi"("error in (no error)"=w127, "Number Samples to Average"=u8 30, "Minimum Rate"=20.0, "EncoderDevRef"=w128) -> ("error out"=w131:errorcluster, "EncoderDevRef"=w132:T38)  [unwired: 6 in]
  n107 = call-poly <vilib>:"WPI_SolenoidSet.vi"("Value"=WPI_SolenoidValue."Off", "SolenoidDevRef"=w108) -> ("SolenoidDevRef"=w107:T35)  [unwired: 8 in, 1 out]
  n108 = disable-structure shown="Disabled" {
    frame Disabled {
      n109 = call <vilib>:"WPI_DigitalInputOpen.vi"("DIO Channel"=FPGA_DIOChannel."DIO 12", "Digital Module (Module 1)"=FPGA_TypedefDigitalModule."Digital Module 1") -> ("error out"=w320:errorcluster, "DigitalInputDevRef"=w321:T19)  [unwired: 8 in]
      n110 = call <vilib>:"WPI_DigitalInputRefNum Registry Set.vi"("error in (no error)"=w320, "refnum name"="alignSwitchLeft", "DigitalInputDevRef"=w321) -> ()  [unwired: 7 in, 2 out]
      n111 = call <vilib>:"WPI_DigitalInputOpen.vi"("DIO Channel"=FPGA_DIOChannel."DIO 13", "Digital Module (Module 1)"=FPGA_TypedefDigitalModule."Digital Module 1") -> ("error out"=w322:errorcluster, "DigitalInputDevRef"=w323:T19)  [unwired: 8 in]
      n112 = call <vilib>:"WPI_DigitalInputRefNum Registry Set.vi"("error in (no error)"=w322, "refnum name"="alignSwitchRight", "DigitalInputDevRef"=w323) -> ()  [unwired: 7 in, 2 out]
    }
    frame Enabled {
    }
  }
  n113 = TDMS Read(0:w69, 1:w63, 5:w71, 7:w70, 11:w66, 12:w12) -> (4:w16:refnum<k34>, 6:w11:string, 10:w17:dbl[], 15:w14:errorcluster)  [unwired: 2 in, 2 out]
  n114 = call <vilib>:"WPI_EncoderStart.vi"("error in (no error)"=w131, "EncoderDevRef"=w132) -> ("error out"=w133:errorcluster, "EncoderDevRef"=w134:T38)  [unwired: 8 in]
  n115 = disable-structure shown="Disabled" {
    frame Disabled {
      (unwired) 0.053884 ("DistancePerCount")
      (unwired) 0.049958 ("DistancePerCount")
    }
    frame Enabled {
    }
  }
  n116 = call <vilib>:"WPI_SolenoidRefNum Registry Set.vi"("refnum name"="pullUp", "SolenoidDevRef"=w107) -> ()  [unwired: 8 in, 2 out]
  n117 = Index Array(array=w17, index=w8) -> (element=w6:dbl)
  n118 = TDMS Read(0:w16, 1:w63, 5:w11, 7:"Right Enc" ("channel name(s) in"), 11:w14, 12:w12) -> (4:w15:refnum<k34>, 10:w9:dbl[], 15:w13:errorcluster)  [unwired: 2 in, 3 out]
  n119 = call <vilib>:"WPI_EncoderRefNum Registry Set.vi"("error in (no error)"=w133, "refnum name"="climbSensor", "EncoderDevRef"=w134) -> ()  [unwired: 7 in, 2 out]
  n120 = call-poly <vilib>:"WPI_SolenoidOpen.vi"("Reverse Solenoid Channel"=WPI_SolenoidChannel."Solenoid 8", "Forward Solenoid Channel"=WPI_SolenoidChannel."Solenoid 7", "Solenoid Module (Module 1)"=FPGA_TypedefSolenoidModule."Solenoid Module 1") -> ("error out"=w35:errorcluster, "SolenoidDevRef"=w34:T35)  [unwired: 7 in]
  n121 = call <vilib>:"WPI_DigitalInputOpen.vi"("DIO Channel"=FPGA_DIOChannel."DIO 5", "Digital Module (Module 1)"=FPGA_TypedefDigitalModule."Digital Module 1") -> ("DigitalInputDevRef"=w50:T19)  [unwired: 8 in, 1 out]
  n122 = call <vilib>:"WPI_GyroOpen.vi"("Analog Channel"=FPGA_AIGyroChannel."AI 1", "Analog Module (Module 1)"=FPGA_TypedefAnalogModuleForGyro."Analog Module 1") -> ("error out"=w80:errorcluster, "GyroDevRef"=w79:T41)  [unwired: 7 in, 1 out]
  n123 = shared-variable ".\\Shared Variables.lvlib\\Sensors.lvlib\\Left Odo"(w6) -> ()  [unwired: 1 in, 1 out]
  n124 = Index Array(array=w9, index=w8) -> (element=w7:dbl)
  n125 = call <vilib>:"WPI_AnalogChannelOpen.vi"("Analog Channel"=FPGA_AIChannel."AI 4", "Analog Module (Module 1)"=FPGA_TypedefAnalogModule."Analog Module 1" ("Analog Module (Slot 1)")) -> ("error out"=w22:errorcluster, "AIDeviceRef"=w23:T36)  [unwired: 1 in, 7 out]
  n126 = TDMS Close(8:w13, 11:w15) -> ()  [unwired: 2 out]
  n127 = call-poly <vilib>:"WPI_SolenoidSet.vi"("error in (no error)"=w35, "Value"=WPI_SolenoidValue."Reverse", "SolenoidDevRef"=w34) -> ("error out"=w32:errorcluster, "SolenoidDevRef"=w31:T35)  [unwired: 7 in]
  n128 = call-poly <vilib>:"WPI_CounterToDigitalSource.vi"("DigitalInputDevRef"=w50) -> ("Digital Source"=w49:T23)  [unwired: 6 in]
  n129 = call <vilib>:"WPI_GyroSetGain.vi"("error in (no error)"=w80, "Gain (VoltsPerDegree/Second)"=0.006611, "GyroDevRef"=w79) -> ("error out"=w77:errorcluster, "GyroDevRef"=w78:T41)  [unwired: 7 in]
  n130 = call <vilib>:"WPI_ServoOpen.vi"("PWM Channel"=FPGA_DIOPWMChannel."PWM 8", "Digital Module (Module 1)"=FPGA_TypedefDigitalModule."Digital Module 1") -> ("error out"=w60:errorcluster, "ServoDeviceRef"=w59:T29)  [unwired: 8 in]
  n131 = shared-variable ".\\Shared Variables.lvlib\\Sensors.lvlib\\Right Odo"(w7) -> ()  [unwired: 1 in, 1 out]
  n132 = call <vilib>:"WPI_AnalogChannelRefNum Registry Set.vi"("error in (no error)"=w22, "refnum name"="Sonar", "AIDeviceRef"=w23) -> ()  [unwired: 9 out]
  n133 = call <vilib>:"WPI_SolenoidRefNum Registry Set.vi"("error in (no error)"=w32, "refnum name"="discSolenoid", "SolenoidDevRef"=w31) -> ()  [unwired: 7 in, 2 out]
  n134 = call <vilib>:"WPI_GyroRefNum Registry Set.vi"("error in (no error)"=w77, "refnum name"="turnGyro", "GyroDevRef"=w78) -> ()  [unwired: 7 in, 2 out]
  n135 = call <vilib>:"WPI_ServoRefNum Registry Set.vi"("error in (no error)"=w60, "refnum name"="loadServoBack", "ServoDeviceRef"=w59) -> ()  [unwired: 7 in, 2 out]
  n136 = call-poly <vilib>:"WPI_CounterOpen.vi"("Source"=w49) -> ("CounterDevRef"=w46:T27)  [unwired: 9 in, 1 out]
  n137 = call <vilib>:"WPI_CounterConfigureTimer.vi"("Number Samples to Average"=u8 2, "MaxPeriod (sec)"=0.25, "CounterDevRef in"=w46) -> ("error out"=w43:errorcluster, "CounterDevRef out"=w42:T27)  [unwired: 7 in]
  n138 = disable-structure shown="Disabled" {
    frame Disabled {
      w326 = "%.;%d.%d.%d.%d" ("format string")
      # "When the camera is plugged into the\nrobot switch, use the robot IP to compute\nthe camera IP address"
      # "Initialize camera settings. You may want to update resolution, or size elsewhere."
      n139 = String To IP() -> (0:w333:u32)  [unwired: 1 in]
      n140 = IP To String(1:TRUE ("dot notation? (F)"), 2:w333) -> (0:w331:string)
      n141 = Scan From String(format string=w326, input string=w331) -> (output 1=w330:i32, output 2=w329:i32, output 3=w328:i32)  [unwired: 7 in, 3 out]
      n142 = Format Into String(format string=w326, w330, w329, w328, 11 ("Compression")) -> (resulting string=w325:string)  [unwired: 2 in, 1 out]
      n143 = call <vilib>:"WPI_CameraOpen.vi"("Camera Address"=w325) -> ("error out"=w345:errorcluster, "CameraDevRef"=w346:T45)  [unwired: 1 in, 8 out]
      n144 = call <vilib>:"WPI_CameraSet Image Size.vi"("error in (no error)"=w345, "Image Size"="Image Size", "CameraDevRef"=w346) -> ("error out"=w344:errorcluster, "CameraDevRef Out"=w347:T45)  [unwired: 7 out]
      n145 = call <vilib>:"WPI_CameraSet Frame Rate.vi"("error in (no error)"=w344, "Frame Rate (fps)"=T42 12, "CameraDevRef"=w347) -> ("error out"=w343:errorcluster, "CameraDevRef Out"=w349:T45)  [unwired: 7 out]
      n146 = call <vilib>:"WPI_CameraSet White Balance.vi"("error in (no error)"=w343, "White Balance"=WPI_CameraWhite_Balance_Values."Fixed fluorescent 1", "CameraDevRef"=w349) -> ("error out"=w342:errorcluster, "CameraDevRef Out"=w348:T45)  [unwired: 7 out]
      n147 = call <vilib>:"WPI_CameraSet Exposure.vi"("error in (no error)"=w342, "Exposure"=WPI_CameraExposure_Values."Auto", "CameraDevRef"=w348) -> ("error out"=w341:errorcluster, "CameraDevRef Out"=w351:T45)  [unwired: 7 out]
      n148 = call <vilib>:"WPI_CameraSet Image Compression.vi"("error in (no error)"=w341, "Compression"=40, "CameraDevRef"=w351) -> ("error out"=w340:errorcluster, "CameraDevRef Out"=w350:T45)  [unwired: 7 out]
      n149 = call <vilib>:"WPI_CameraSet Brightness.vi"("error in (no error)"=w340, "Brightness"=50, "CameraDevRef"=w350) -> ("error out"=w338:errorcluster, "CameraDevRef Out"=w339:T45)  [unwired: 7 out]
      n150 = call <vilib>:"WPI_CameraRefNum Registry Set.vi"("error in (no error)"=w338, "refnum name"="Camera", "CameraDevRef"=w339) -> ("error out"=w324:errorcluster)  [unwired: 8 out]
    }
    frame Enabled {
    }
  }
  n151 = call <vilib>:"WPI_CounterStart.vi"("error in (no error)"=w43, "CounterDevRef in"=w42) -> ("error out"=w41:errorcluster, "CounterDevRef out"=w40:T27)  [unwired: 8 in]
  n152 = call <vilib>:"WPI_CounterRefNum Registry Set.vi"("error in (no error)"=w41, "refnum name"="shooterRpm", "CounterDevRef"=w40) -> ()  [unwired: 7 in, 2 out]
  "error out" <- errorcluster {"status"=FALSE, "code"=0, "source"=""} ("error out")
